vi "lectura de angulos de euler.vi"(4 "read buffer":string) -> (0 "Yaw":i32[](array[numeric]), 1 "Pitch":i32[](array[numeric]), 2 "Roll":i32[](array[numeric]))   [LabVIEW 2018]
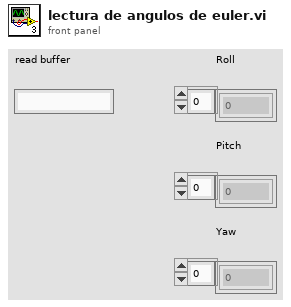
[diagram p1: front panel]
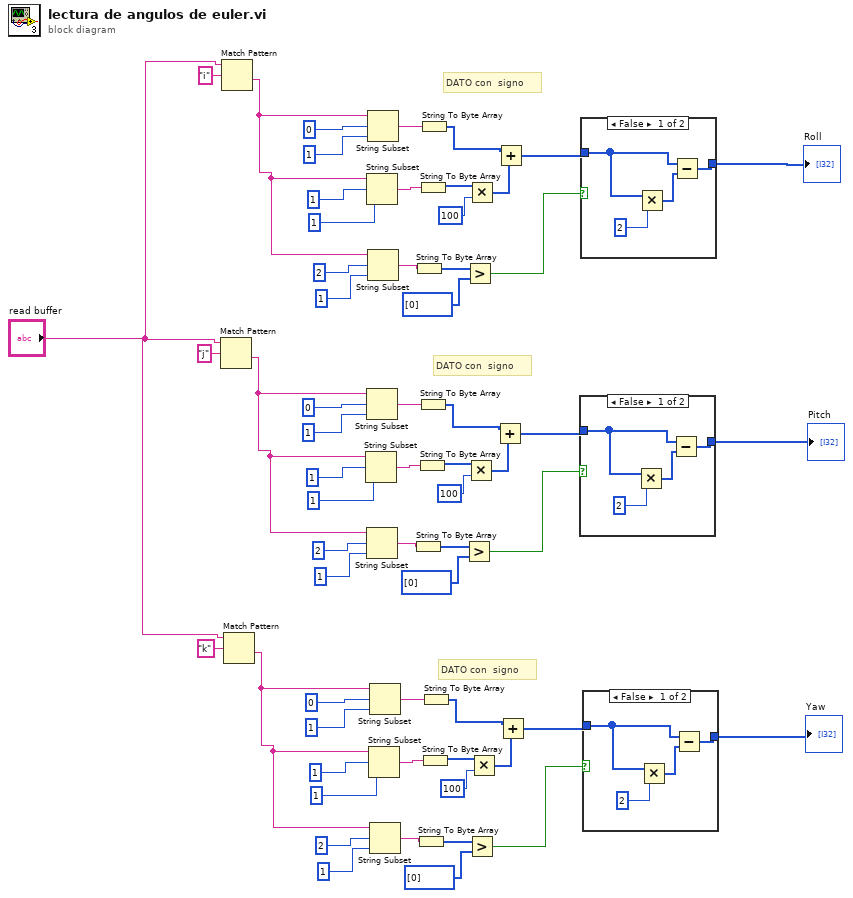
[diagram p0: block diagram]
diagram:
  # "DATO con  signo"
  # "DATO con  signo"
  # "DATO con  signo"
  n1 = Match Pattern(string="read buffer", regular expression="j") -> (after substring=w39:string)  [unwired: 1 in, 3 out]
  n2 = Match Pattern(string="read buffer", regular expression="i") -> (after substring=w19:string)  [unwired: 1 in, 3 out]
  n3 = Match Pattern(string="read buffer", regular expression="k") -> (after substring=w59:string)  [unwired: 1 in, 3 out]
  n4 = String Subset(string=w39, offset (0)=1, length (rest)=1 ("length (rest)")) -> (substring=w29:string)
  n5 = String Subset(string=w19, offset (0)=1, length (rest)=1 ("length (rest)")) -> (substring=w9:string)
  n6 = String Subset(string=w39, offset (0)=0, length (rest)=1 ("length (rest)")) -> (substring=w30:string)
  n7 = String Subset(string=w39, offset (0)=2, length (rest)=1 ("length (rest)")) -> (substring=w24:string)
  n8 = String Subset(string=w19, offset (0)=0, length (rest)=1 ("length (rest)")) -> (substring=w10:string)
  n9 = String Subset(string=w19, offset (0)=2, length (rest)=1 ("length (rest)")) -> (substring=w4:string)
  n10 = String Subset(string=w59, offset (0)=1, length (rest)=1 ("length (rest)")) -> (substring=w49:string)
  n11 = String Subset(string=w59, offset (0)=0, length (rest)=1 ("length (rest)")) -> (substring=w50:string)
  n12 = String Subset(string=w59, offset (0)=2, length (rest)=1 ("length (rest)")) -> (substring=w44:string)
  n13 = String To Byte Array(string=w24) -> (unsigned byte array=w23:u8[])
  n14 = String To Byte Array(string=w4) -> (unsigned byte array=w3:u8[])
  n15 = String To Byte Array(string=w44) -> (unsigned byte array=w43:u8[])
  n16 = String To Byte Array(string=w29) -> (unsigned byte array=w28:u8[])
  n17 = String To Byte Array(string=w9) -> (unsigned byte array=w8:u8[])
  n18 = String To Byte Array(string=w30) -> (unsigned byte array=w25:u8[])
  n19 = String To Byte Array(string=w10) -> (unsigned byte array=w5:u8[])
  n20 = String To Byte Array(string=w49) -> (unsigned byte array=w48:u8[])
  n21 = String To Byte Array(string=w50) -> (unsigned byte array=w45:u8[])
  n22 = Greater?(x=w23, y=u8[] [0]) -> (0:w21:bool)
  n23 = Greater?(x=w3, y=u8[] [0]) -> (0:w1:bool)
  n24 = Multiply(x=w28, y=100) -> (x*y=w26:i32[])
  n25 = Multiply(x=w8, y=100) -> (x*y=w6:i32[])
  n26 = Greater?(x=w43, y=u8[] [0]) -> (0:w41:bool)
  n27 = Multiply(x=w48, y=100) -> (x*y=w46:i32[])
  n28 = Add(x=w25, y=w26) -> (x+y=w37:i32[])
  n29 = Add(x=w5, y=w6) -> (x+y=w17:i32[])
  n30 = Add(x=w45, y=w46) -> (x+y=w57:i32[])
  n31 = case shown="False" w21 {
    tunnel: w37 -> [w64 w66]
    tunnel: [w63 w66] -> w40
    frame False {
      n32 = Multiply(x=w64, y=2) -> (x*y=w65:i32[])
      n33 = Subtract(x=w64, y=w65) -> (x-y=w63:i32[])
    }
    frame True {
    }
  }
  "Pitch" <- w40
  n34 = case shown="False" w1 {
    tunnel: w17 -> [w69 w71]
    tunnel: [w68 w71] -> w20
    frame False {
      n35 = Multiply(x=w69, y=2) -> (x*y=w70:i32[])
      n36 = Subtract(x=w69, y=w70) -> (x-y=w68:i32[])
    }
    frame True {
    }
  }
  "Roll" <- w20
  n37 = case shown="False" w41 {
    tunnel: w57 -> [w74 w76]
    tunnel: [w73 w76] -> w60
    frame False {
      n38 = Multiply(x=w74, y=2) -> (x*y=w75:i32[])
      n39 = Subtract(x=w74, y=w75) -> (x-y=w73:i32[])
    }
    frame True {
    }
  }
  "Yaw" <- w60
